vi "Do.vi"(8 "error in":errorcluster, 10 "Actor in":refnum<class "Actor.lvclass">, 11 "Ship Wvfm Data MSG":refnum<class "Ship Wvfm Data MSG.lvclass">) -> (0 "error out":errorcluster, 2 "Actor out":refnum<class "Actor.lvclass">)   [LabVIEW 2014, in "ePAS Library.lvlib" / "Ship Wvfm Data MSG.lvclass"]
doc: "(<B>Filename</B>: Actor Framework.lvlib:Message.lvclass:Do.vi)\n\nDefines what a message does when it is received by an actor. Generally, a message instructs an actor to invoke one of its methods. By default, this method does nothing. A child class must override it to define behavior. Create a child class by using the Actor Framework Message Maker dialog box."
uses:
  Ship Wvfm Data MSG.lvclass
  <vilib>/ActorFramework/Actor/Actor.lvclass
  Ship Wvfm Data MSG.lvclass/Ship Wvfm Data MSG.ctl
  Instr Actor/Instr Actor.lvclass
  Commands/Set Wvfm Write/Set Wvfm Write CMD.lvclass
  Commands/Set Wvfm Write/Set Wvfm Write CMD.lvclass/Set Wvfm Write CMD.ctl
  SuperActor/Ex Nested.lvclass/Ex Nested.ctl
  SuperActor/Read CVT Session.vi
  SuperActor/Read Log Session.vi
  Commands/Set Wvfm Write/Write Write_.vi
  <userlib>/_Session Fwk/Session - Root.lvclass
  reusable/Command/Command.lvclass
  reusable/Session APIs/Session Log/System Log.lvclass
  reusable/Session APIs/CVT/CVT.lvclass
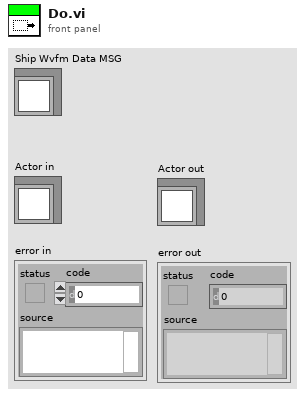
[diagram p1: front panel]
types:
  T1 = typedef "Session - Root.lvclass/Session Handle.ctl" = refnum<data-value>
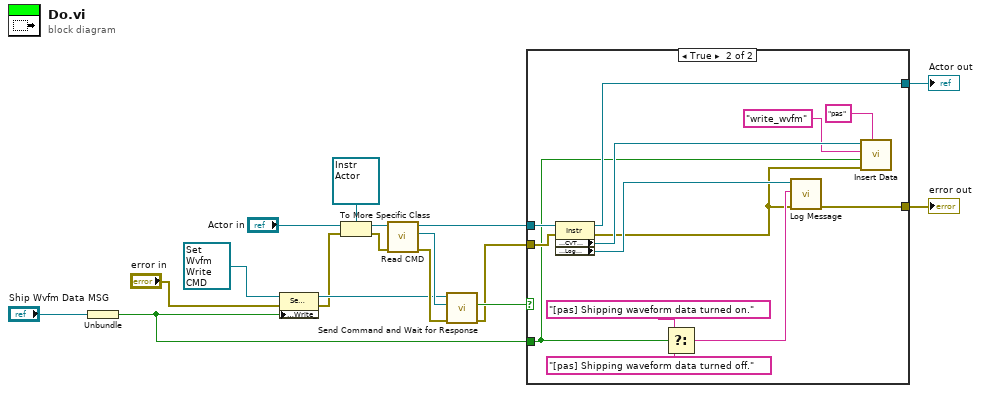
[diagram p0: block diagram]
diagram:
  n1 = Unbundle("Ship Wvfm Data MSG") -> (w1:bool)
  n2 = property class="Set Wvfm Write CMD"(reference=refnum<class "Set Wvfm Write CMD.lvclass"> refnum ("ePAS Library.lvlib:Set Wvfm Write CMD"), error in="error in", "Accessors:Write_"=w1) -> (reference out=w7:refnum<class "Set Wvfm Write CMD.lvclass">, error out=w4:errorcluster)
  n3 = To More Specific Class(target class=refnum<class "Instr Actor.lvclass"> refnum ("Instrument Lib:Instr"), reference="Actor in", error in=w4) -> (specific class reference=w3:refnum<class "Instr Actor.lvclass">, error out=w16:errorcluster)
  n4 = call "Read CMD.vi"("error in (no error)"=w16, "Instr Actor in"=w3) -> ("error out"=w15:errorcluster, "CMD"=w14:refnum<queue>, "Instr Actor out"=w10:refnum<class "Instr Actor.lvclass">)  [unwired: 7 in]
  n5 = call "Send Command and Wait for Response.vi"("error in"=w15, "cmd queue"=w14, "CMD in"=w7) -> ("error out"=w12:errorcluster, "cmd good?"=w13:bool)  [unwired: 6 in, 1 out]
  n6 = case shown="True" w13 {
    tunnel: w10 -> [w19 w32]
    tunnel: [w19 w31] -> w2
    tunnel: w12 -> [w18 w26]
    tunnel: [w18 w20] -> w9
    tunnel: w1 -> [_ w22]
    frame False {
    }
    frame True {
      n7 = property class="Instr"(reference=w32, error in=w26) -> (reference out=w31:refnum<class "Instr Actor.lvclass">, error out=w21:errorcluster, "Accessors:CVT Session"=w25:T1, "Accessors:Log Session"=w30:T1)
      n8 = Select(t="[pas] Shipping waveform data turned on." ("MSG In"), s=w22, f="[pas] Shipping waveform data turned off." ("MSG In")) -> (s? t:f=w27:string)
      n9 = call "Log Message.vi"("error in"=w21, "MSG In"=w27, "session in"=w30) -> ("error out"=w20:errorcluster)  [unwired: 7 in, 1 out]
      n10 = call "Insert Data.vi"("Group"="pas", "error in"=w21, "Data"=w22, "tag"="write_wvfm", "CVT Session In"=w25) -> ()  [unwired: 5 in, 2 out]
    }
  }
  "error out" <- w9
  "Actor out" <- w2
